vi "init.vi"(8 "error in (no error)":errorcluster, 11 "ComponentData in":refnum<class "ComponentData.lvclass">) -> (0 "error out":errorcluster, 3 "ComponentData out":refnum<class "ComponentData.lvclass">)   [LabVIEW 2013, in "ComponentData.lvlib" / "ComponentData.lvclass"]
doc: "The configurationTabUI input is needed for Windows, but not VxWorks."
uses:
  <userlib>/Common/Component/Application/RT/ComponentData/ComponentData/ComponentData.lvclass
  <userlib>/Common/Component/Application/RT/ComponentData/ComponentData/ComponentData.lvclass/ComponentData.ctl
  <userlib>/Common/Component/Application/RT/ComponentData/IRQHandler/IRQHandler.lvclass
  <userlib>/Common/Component/Application/RT/ComponentData/LoopTimer/LoopTimer.lvclass
  <userlib>/Common/Component/Application/RT/ComponentData/RIOHandler/RIOHandler.lvclass
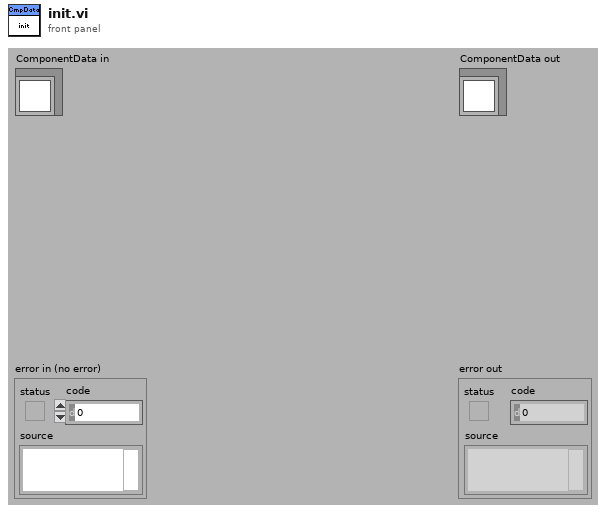
[diagram p1: front panel]
types:
  T1 = enum32{"invalid OS target", "Mac OS", "Windows 3.1", "Windows 95/NT", "Solaris 1", "Solaris 2", "HP-UX", "PowerMAX", "Linux", "Irix", "Rhapsody", "BeOS", "AIX", "OSF1", "VxWorks", "PharLap", "Carbon", "RTX", "Windows x64", "Linux x64"}
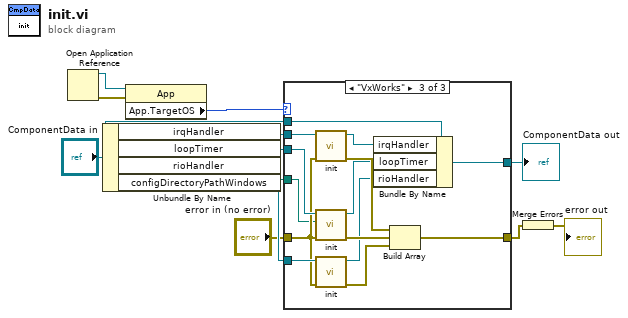
[diagram p0: block diagram]
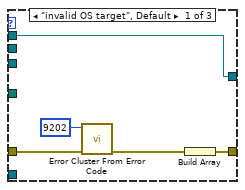
[diagram p2: hidden frame]
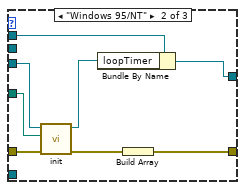
[diagram p3: hidden frame]
diagram:
  n1 = Open Application Reference() -> (0:w5:errorcluster, 3:w6:refnum<vi>)  [unwired: 4 in]
  n2 = Unbundle By Name("ComponentData in") -> ("irqHandler"=w12:refnum<class "IRQHandler.lvclass">, "loopTimer"=w10:refnum<class "LoopTimer.lvclass">, "rioHandler"=w9:refnum<class "RIOHandler.lvclass">, "configDirectoryPathWindows"=w7:path)
  n3 = property class="App"(reference=w6, error in=w5) -> ("App.TargetOS"=w4:T1)  [unwired: 2 out]
  n4 = case shown="\"VxWorks\"" w4 {
    tunnel: w12 -> [_ _ w39]
    tunnel: w10 -> [_ w25 w38]
    tunnel: w9 -> [_ _ w37]
    tunnel: "error in (no error)" -> [w15 w24 w36]
    tunnel: w7 -> [_ w23 w35]
    tunnel: [w16 w21 w26] -> w3
    tunnel: "ComponentData in" -> [w17 w20 w28]
    tunnel: [w17 w18 w27] -> w1
    frame "invalid OS target", Default {
      n5 = call <vilib>:"Error Cluster From Error Code.vi"("error in (no error)"=w15, "error code (0)"=9202) -> ("error out"=w14:errorcluster)  [unwired: 7 in]
      n6 = Build Array(w14) -> (w16:errorcluster[])
    }
    frame "Windows 95/NT" {
      n7 = call <userlib>:"init.vi"("error in (no error)"=w24, "configDirectoryPathWindows"=w23, "LoopTimer in"=w25) -> ("error out"=w22:errorcluster, "LoopTimer out"=w19:refnum<class "LoopTimer.lvclass">)  [unwired: 7 in]
      n8 = Bundle By Name(cluster=w20, "loopTimer"=w19) -> (w18:refnum<class "ComponentData.lvclass">)
      n9 = Build Array(w22) -> (w21:errorcluster[])
    }
    frame "VxWorks" {
      n10 = call <userlib>:"init.vi"("error in (no error)"=w36, "IRQHandler in"=w39) -> ("error out"=w34:errorcluster, "IRQHandler out"=w31:refnum<class "IRQHandler.lvclass">)  [unwired: 8 in]
      n11 = call <userlib>:"init.vi"("error in (no error)"=w36, "configDirectoryPathWindows"=w35, "LoopTimer in"=w38) -> ("error out"=w33:errorcluster, "LoopTimer out"=w30:refnum<class "LoopTimer.lvclass">)  [unwired: 7 in]
      n12 = call <userlib>:"init.vi"("error in (no error)"=w36, "RIOHandler in"=w37) -> ("error out"=w32:errorcluster, "RIOHandler out"=w29:refnum<class "RIOHandler.lvclass">)  [unwired: 8 in]
      n13 = Bundle By Name(cluster=w28, "irqHandler"=w31, "loopTimer"=w30, "rioHandler"=w29) -> (w27:refnum<class "ComponentData.lvclass">)
      n14 = Build Array(w34, w33, w32) -> (w26:errorcluster[])
    }
  }
  "ComponentData out" <- w1
  n15 = Merge Errors(w3) -> (→"error out":errorcluster)
